vi "Pockels Cal_Resize output array.vi"(10 "Numeric":i32, 11 "Loaded cal file":string[][](array[string])) -> (3 "Array":string[][](array[string]))   [LabVIEW 2013]
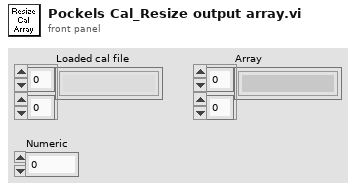
[diagram p1: front panel]
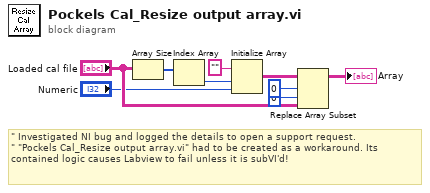
[diagram p0: block diagram]
diagram:
  # "\"\tInvestigated NI bug and logged the details to open a support request.\n\"\t\"Pockels Cal_Resize output array.vi\" had to be created as a workaround. Its contained logic causes Labview to fail unless it is subVI'd!"
  n1 = Array Size(array="Loaded cal file") -> (size(s)=w6:i32[])
  n2 = Index Array(array=w6) -> (element=w5:i32)  [unwired: 1 in]
  n3 = Initialize Array("" ("element"), w5, "Numeric") -> (w3:string[][])
  n4 = Replace Array Subset "Replace Array Subset"(array=w3, new element="Loaded cal file", index (row)=0, index (col)=0 ("disabled index (col)")) -> (→"Array":string[][])
